vi "MB ICPCON Param Write timeouts.vi"(8 "error in (no error)":errorcluster, 9 "timeouts":T1[](array[typedef]), 10 "index (0)":i32, 11 "Param Reference":T2) -> (0 "error out":errorcluster, 3 "Param Reference out":T2)   [LabVIEW 2019, in "ICPCON_Param.lvlib"]
uses:
  ICPCON_Param.lvlib
  ICPCON Param.ctl
  Eth timeouts.ctl
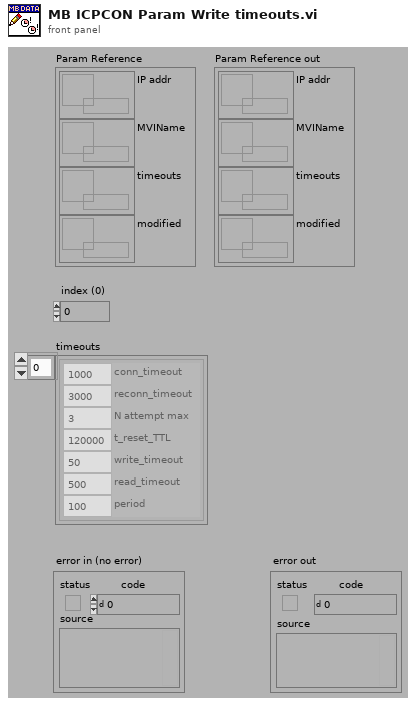
[diagram p1: front panel]
types:
  T1 = typedef "ICPCON_Param.lvlib/Eth timeouts.ctl" = cluster{"conn_timeout":i32, "reconn_timeout":i32, "N attempt max":i32, "t_reset_TTL":i32, "write_timeout":i32, "read_timeout":i32, "period":i32}
  T2 = typedef "ICPCON_Param.lvlib/ICPCON Param.ctl" = cluster{"IP addr":refnum<data-value>, "MVIName":refnum<data-value>, "timeouts":refnum<data-value>, "modified":refnum<data-value>}
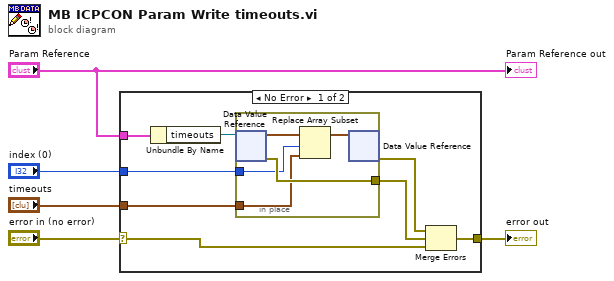
[diagram p0: block diagram]
diagram:
  n1 = case shown="No Error" "error in (no error)" {
    selector: "error in (no error)" -> [w6 w19]
    tunnel: [w11 w19] -> w4
    tunnel: "index (0)" -> [w13 _]
    tunnel: "Param Reference" -> [w12 _]
    tunnel: "timeouts" -> [w10 _]
    frame No Error {
      n2 = Unbundle By Name(w12) -> ("timeouts"=w7:refnum<data-value>)
      n3 = in-place {
        in-place-border: w13 -> [w15]
        in-place-border: [w18] -> w8
        in-place-border: w10 -> [w14]
        n4 = in-place-dvr #1(w7) -> (w17:T1[], w18:errorcluster)
        n5 = Replace Array Subset(array=w17, new element=w14, index=w15) -> (w16:T1[])
        n6 = in-place-dvr #1(w16) -> (w9:errorcluster)  [unwired: 1 out]
      }
      n7 = Merge Errors(w9, w8, w6) -> (w11:errorcluster)
    }
    frame Error {
    }
  }
  "error out" <- w4
  "Param Reference out" <- "Param Reference"
